vi "ErrorLog.vi"(2 "error in":errorcluster, 3 "String in":string, 4 "Error String":string) -> (0 "Success?":bool, 1 "String out":string)   [LabVIEW 2010]
uses:
  <vilib>/Utility/error.llb/DialogType.ctl
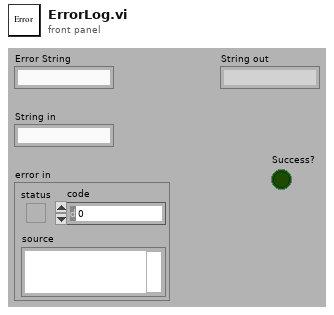
[diagram p1: front panel]
types:
  T1 = typedef "DialogType.ctl" = u16
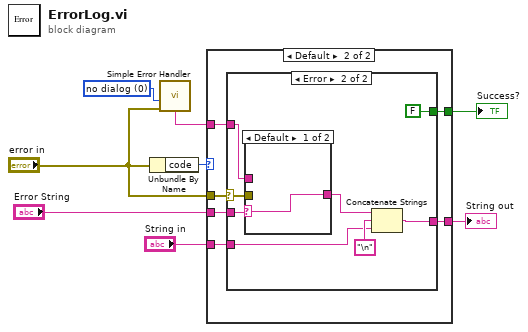
[diagram p0: block diagram]
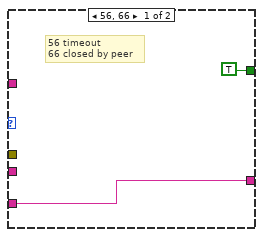
[diagram p2: hidden frame]
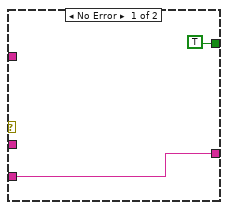
[diagram p3: hidden frame]
diagram:
  w6 = T1 0 items=["no dialog", "OK message", "continue or stop message", "OK message + warnings", "continue/stop + warnings"] ("type of dialog (OK msg:1)")
  n1 = Unbundle By Name("error in") -> ("code"=w3:i32)
  n2 = call <vilib>:"Simple Error Handler.vi"("type of dialog (OK msg:1)"=w6, "error in (no error)"="error in") -> ("message"=w2:string)  [unwired: 3 in, 4 out]
  n3 = case shown="Default" w3 {
    tunnel: "Error String" -> [_ w16]
    tunnel: [w10 w15] -> w7
    tunnel: "String in" -> [w10 w14]
    tunnel: "error in" -> [_ w13]
    tunnel: w2 -> [_ w12]
    tunnel: [TRUE w11] -> w1
    frame 56, 66 {
      # "56 timeout\n66 closed by peer"
    }
    frame Default {
      n4 = case shown="Error" w13 {
        selector: w13 -> [_ w23]
        tunnel: w16 -> [_ w24]
        tunnel: [w18 w26] -> w15
        tunnel: w14 -> [w18 w20]
        tunnel: w12 -> [_ w22]
        tunnel: [TRUE FALSE] -> w11
        frame No Error {
        }
        frame Error {
          n5 = case shown="Default" w24 {
            selector: w24 -> [w27 _]
            tunnel: w23 -> [_ _]
            tunnel: [w27 w28] -> w21
            tunnel: w22 -> [_ w28]
            frame Default {
            }
            frame "" {
            }
          }
          n6 = Concatenate Strings(w21, "\n" ("string"), w20) -> (w26:string)
        }
      }
    }
  }
  "String out" <- w7
  "Success?" <- w1
